vi "ChooseCowlState.vi"(0 "Distance (in)":dbl) -> (1 "Desired State":string)   [LabVIEW 2019]
doc: "This VI decides which cowl position should be used based on the current ranging information."
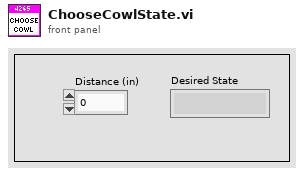
[diagram p1: front panel]
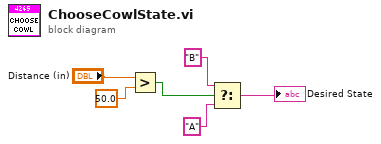
[diagram p0: block diagram]
diagram:
  n1 = Greater?(x="Distance (in)", y=50.0) -> (0:w3:bool)
  n2 = Select(t="B", s=w3, f="A") -> (s? t:f=→"Desired State":string)
